vi "Status State.vi"(4 "Status State In":string, 5 "Write":bool) -> (1 "Status State Out":string)   [LabVIEW 2019]
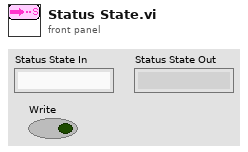
[diagram p1: front panel]
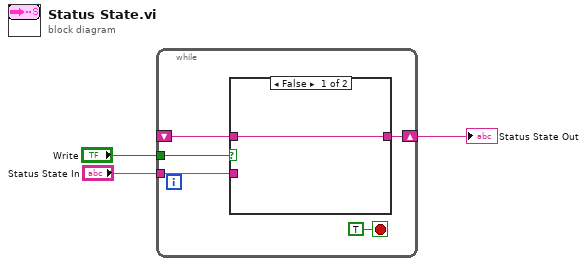
[diagram p0: block diagram]
diagram:
  n1 = while {
    tunnel: "Status State In" -> [w6]
    shift-right: [w7] -> w2
    shift-left: _ -> [w5]
    tunnel: "Write" -> [w4]
    stop <- TRUE stop-if-true
    n2 = case shown="False" w4 {
      tunnel: [w9 w10] -> w7
      tunnel: w6 -> [_ w10]
      tunnel: w5 -> [w9 _]
      frame False {
      }
      frame True {
      }
    }
  }
  "Status State Out" <- w2
